vi "Test Cryogen Levels.vi"(8 "warningcontN":T1, 9 "warningcontHe":T2, 10 "LNlevel":dbl, 11 "LHelevel":dbl) -> (1 "warnN":bool, 2 "warnHe":bool, 3 "warning":T3)   [LabVIEW 2017, in "Level Meter.lvclass"]
uses:
  Level Meter.lvclass
  Level Meter.lvclass/Level Meter.ctl
panel:
  out "Level Meter out":refnum<class "Level Meter.lvclass">
  in  "Level Meter in":refnum<class "Level Meter.lvclass">
  out "error out":errorcluster
  in  "error in (no error)":errorcluster
  # "Off"
  # "On"
  # "Greater"
  # "Less"
  # "Off"
  # "On"
  # "Greater"
  # "Less"
  # "Slow"
  # "Fast"
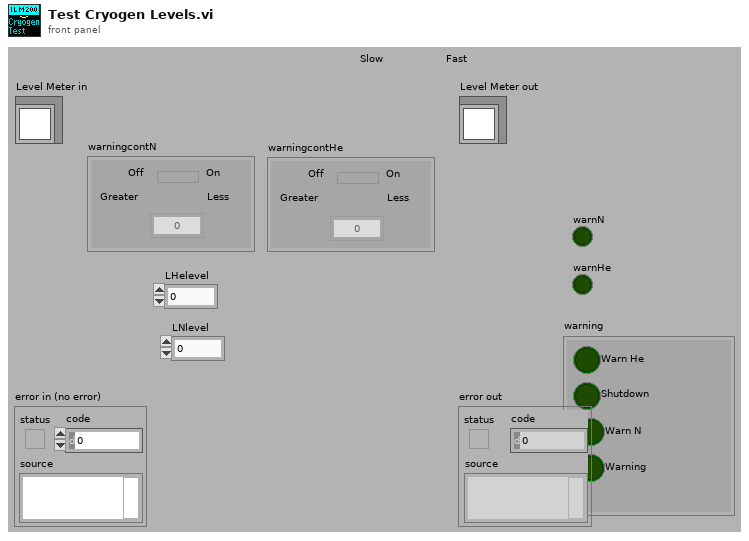
[diagram p1: front panel]
types:
  T1 = cluster{"alarmliqN":dbl, "warn?":bool, "lessthan?":bool}
  T2 = cluster{"alarmliqHe":dbl, "warn?":bool, "lessthan?":bool}
  T3 = cluster{"shutdown?":bool, "warnHe":bool, "warnN":bool, "warn":bool}
  T4 = typedef "OxfordAddress.ctl" = cluster{"Com Port":i32, "ISOBUS Address":i32, "GPIB Address":i16, "Communication":enum16{"RS232", "ISOBUS", "GPIB", "Gateway"}}
  T5 = typedef "ILMRelayStatus.ctl" = cluster{"Shut down":bool, "Alarm sound":bool, "Alarm state":bool, "Silence prohib":bool, "Relay1 active":bool, "Relay 2 active":bool, "Relay 3 active":bool, "Relay 4 active":bool}
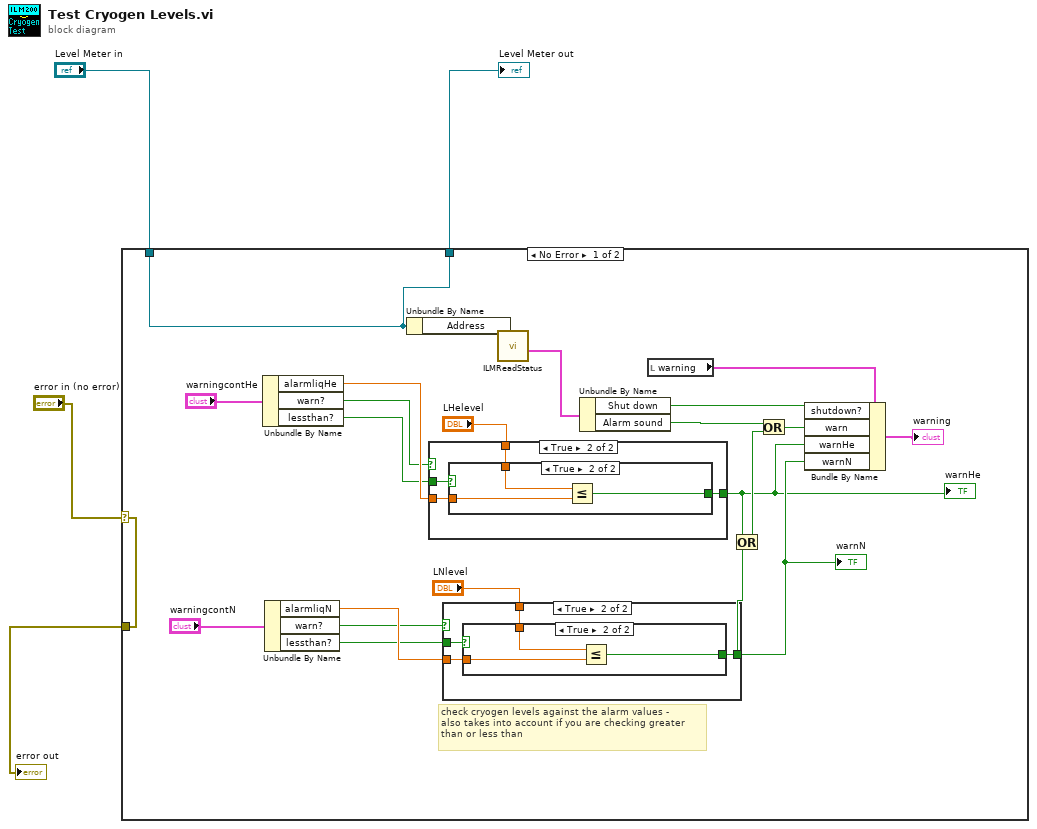
[diagram p0: block diagram]
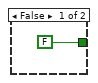
[diagram p2: hidden frame]
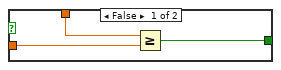
[diagram p3: hidden frame]
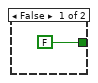
[diagram p4: hidden frame]
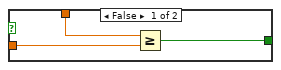
[diagram p5: hidden frame]
diagram:
  n1 = case shown="No Error" "error in (no error)" {
    selector: "error in (no error)" -> [w6 w49]
    tunnel: "Level Meter in" -> [w5 w50]
    tunnel: [w5 w50] -> w2
    tunnel: [w6 w49] -> w1
    frame No Error {
      # "check cryogen levels against the alarm values -\nalso takes into account if you are checking greater\nthan or less than"
      n2 = Unbundle By Name("warningcontHe") -> ("alarmliqHe"=w23:dbl, "warn?"=w21:bool, "lessthan?"=w20:bool)
      n3 = Unbundle By Name("warningcontN") -> ("alarmliqN"=w19:dbl, "warn?"=w18:bool, "lessthan?"=w17:bool)
      n4 = Unbundle By Name(w5) -> ("Address"=w7:T4)
      n5 = case shown="True" w21 {
        tunnel: w20 -> [_ w42]
        tunnel: "LHelevel" -> [_ w39]
        tunnel: w23 -> [_ w41]
        tunnel: [FALSE w40] -> w13
        frame False {
        }
        frame True {
          n6 = case shown="True" w42 {
            tunnel: w41 -> [w44 w47]
            tunnel: [w43 w46] -> w40
            tunnel: w39 -> [w45 w48]
            frame False {
              n7 = Greater Or Equal?(x=w45, y=w44) -> (x >= y?=w43:bool)
            }
            frame True {
              n8 = Less Or Equal?(x=w48, y=w47) -> (x <= y?=w46:bool)
            }
          }
        }
      }
      "warnHe" <- w13
      n9 = case shown="True" w18 {
        tunnel: w17 -> [_ w31]
        tunnel: "LNlevel" -> [_ w28]
        tunnel: w19 -> [_ w30]
        tunnel: [FALSE w29] -> w16
        frame False {
        }
        frame True {
          n10 = case shown="True" w31 {
            tunnel: w30 -> [w33 w36]
            tunnel: [w32 w35] -> w29
            tunnel: w28 -> [w34 w37]
            frame False {
              n11 = Greater Or Equal?(x=w34, y=w33) -> (x >= y?=w32:bool)
            }
            frame True {
              n12 = Less Or Equal?(x=w37, y=w36) -> (x <= y?=w35:bool)
            }
          }
        }
      }
      "warnN" <- w16
      n13 = call "ILMReadStatus.vi"("Instrument address"=w7) -> ("Relay"=w8:T5)  [unwired: 6 out]
      n14 = Unbundle By Name(w8) -> ("Shut down"=w10:bool, "Alarm sound"=w9:bool)
      n15 = local read "warning"() -> (w26:T3)
      n16 = Or(x=w13, y=w16) -> (x .or. y?=w14:bool)
      n17 = Or(x=w9, y=w14) -> (x .or. y?=w15:bool)
      n18 = Bundle By Name(cluster=w26, "shutdown?"=w10, "warn"=w15, "warnHe"=w13, "warnN"=w16) -> (→"warning":T3)
    }
    frame Error {
    }
  }
  "Level Meter out" <- w2
  "error out" <- w1
